vi "SUB_Flush_TxRx_COM.vi"(1 "VISA resource name":refnum<visa-resource-name>) -> ()   [LabVIEW 2011]
uses:
  <vilib>/Instr/_visa.llb/VISA Flush IO Buffer Mask.ctl
  <vilib>/Instr/_visa.llb/Select Event Type.ctl
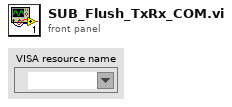
[diagram p1: front panel]
types:
  T1 = typedef "Select Event Type.ctl" = u32
  T2 = typedef "VISA Flush IO Buffer Mask.ctl" = u16
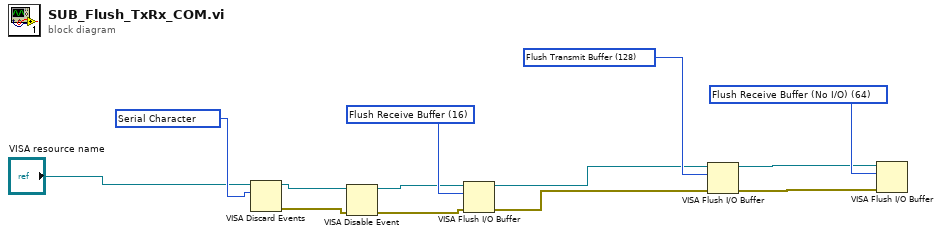
[diagram p0: block diagram]
diagram:
  w3 = T1 1073684533 items=["Service Request"=1073684491, "Trigger"=3221168138, "Clear"=1073684493, "VXI Signal"=1073684512, "VXI/VME Interrupt"=3221168161, "VXI/VME Sysfail"=1073684509, "VXI/VME Sysreset"=1073684510, "GPIB CIC"=1073684498, "GPIB Talk"=1073684499, "GPIB Listen"=1073684500, "PXI Interrupt"=1073684514, "Serial Break"=1073684515, "Serial TermChar"=1073684516, "Serial CTS"=1073684521, "Serial DSR"=1073684522, "Serial DCD"=1073684524, "Serial RI"=1073684526, "Serial Character"=1073684533, "USB Interrupt"=1073684535, "All Enabled"=1073709055] ("Event Type")
  w9 = T2 16 items=["Flush Receive Buffer"=16, "Write Transmit Buffer to Device"=32, "Flush Receive Buffer (No I/O)"=64, "Flush Transmit Buffer"=128] ("Mask")
  w12 = T2 64 items=["Flush Receive Buffer"=16, "Write Transmit Buffer to Device"=32, "Flush Receive Buffer (No I/O)"=64, "Flush Transmit Buffer"=128] ("Mask")
  w13 = T2 128 items=["Flush Receive Buffer"=16, "Write Transmit Buffer to Device"=32, "Flush Receive Buffer (No I/O)"=64, "Flush Transmit Buffer"=128] ("Mask")
  n1 = VISA Discard Events(10:w3, 11:"VISA resource name") -> (0:w1:errorcluster, 3:w6:refnum<visa-resource-name>)  [unwired: 2 in]
  n2 = VISA Disable Event(8:w1, 11:w6) -> (0:w4:errorcluster, 3:w5:refnum<visa-resource-name>)  [unwired: 2 in]
  n3 = VISA Flush I/O Buffer(VISA resource name=w5, mask (16)=w9, error in (no error)=w4) -> (VISA resource name out=w8:refnum<visa-resource-name>, error out=w7:errorcluster)
  n4 = VISA Flush I/O Buffer(VISA resource name=w8, mask (16)=w13, error in (no error)=w7) -> (VISA resource name out=w11:refnum<visa-resource-name>, error out=w10:errorcluster)
  n5 = VISA Flush I/O Buffer(VISA resource name=w11, mask (16)=w12, error in (no error)=w10) -> ()  [unwired: 2 out]
